vi "Examine clusters.vi"(10 "Cluster centers":string[](array[string]), 11 "Pattern (0) Distance data (1 to X) cluster (X+1) output":string[][](array[string])) -> (1 "position counts":T1[](array[typedef]), 2 "Cluster center graph":cluster{"XY Graph":cluster{dbl[], dbl[]}}[](array[cluster]), 3 "Cluster graph":cluster{"XY Graph":cluster{dbl[], dbl[]}[]}[](array[cluster]))   [LabVIEW 2013]
uses:
  cluster.ctl
panel:
  out "Array 2":dbl[](array[numeric])
  out "Cluster":T2
  out "XY Graph 4":cluster{dbl[], dbl[]}(graph)
  in  "XY Graph 6":cluster{dbl[], dbl[]}(graph)
  out "array 2":dbl[][][](array[numeric])
  in  "XY Graph 3":cluster{dbl[], dbl[]}[](graph)
  out "XY Graph":cluster{"X":dbl[], "Y":dbl[]}(graph)
  out "XY Graph 2":cluster{dbl[], dbl[]}[](graph)
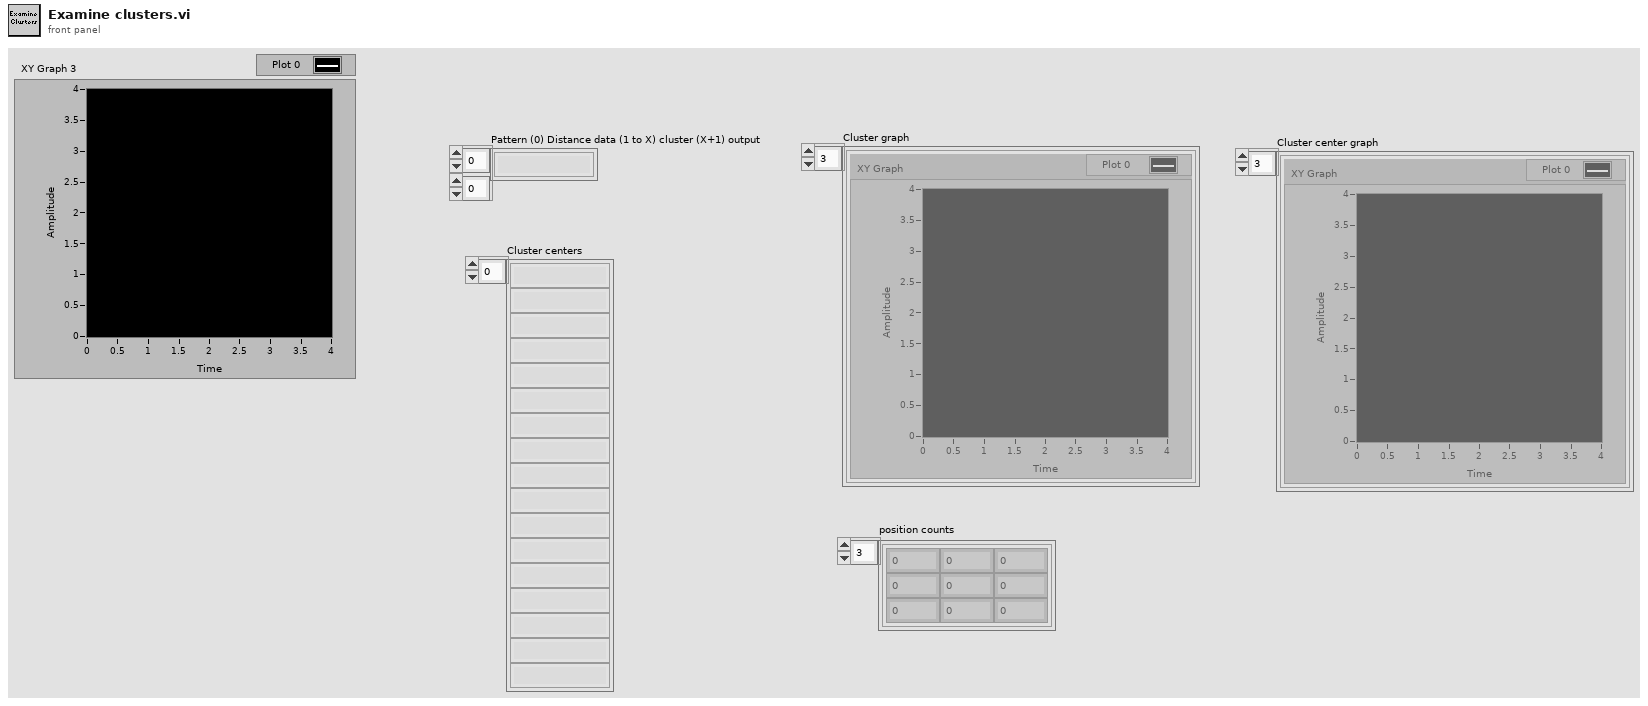
[diagram p1: front panel]
types:
  T1 = typedef "cluster.ctl" = cluster{dbl, dbl, dbl, dbl, dbl, dbl, dbl, dbl, dbl}
  T2 = cluster{dbl, dbl, dbl, dbl, dbl, dbl, dbl, dbl, dbl}
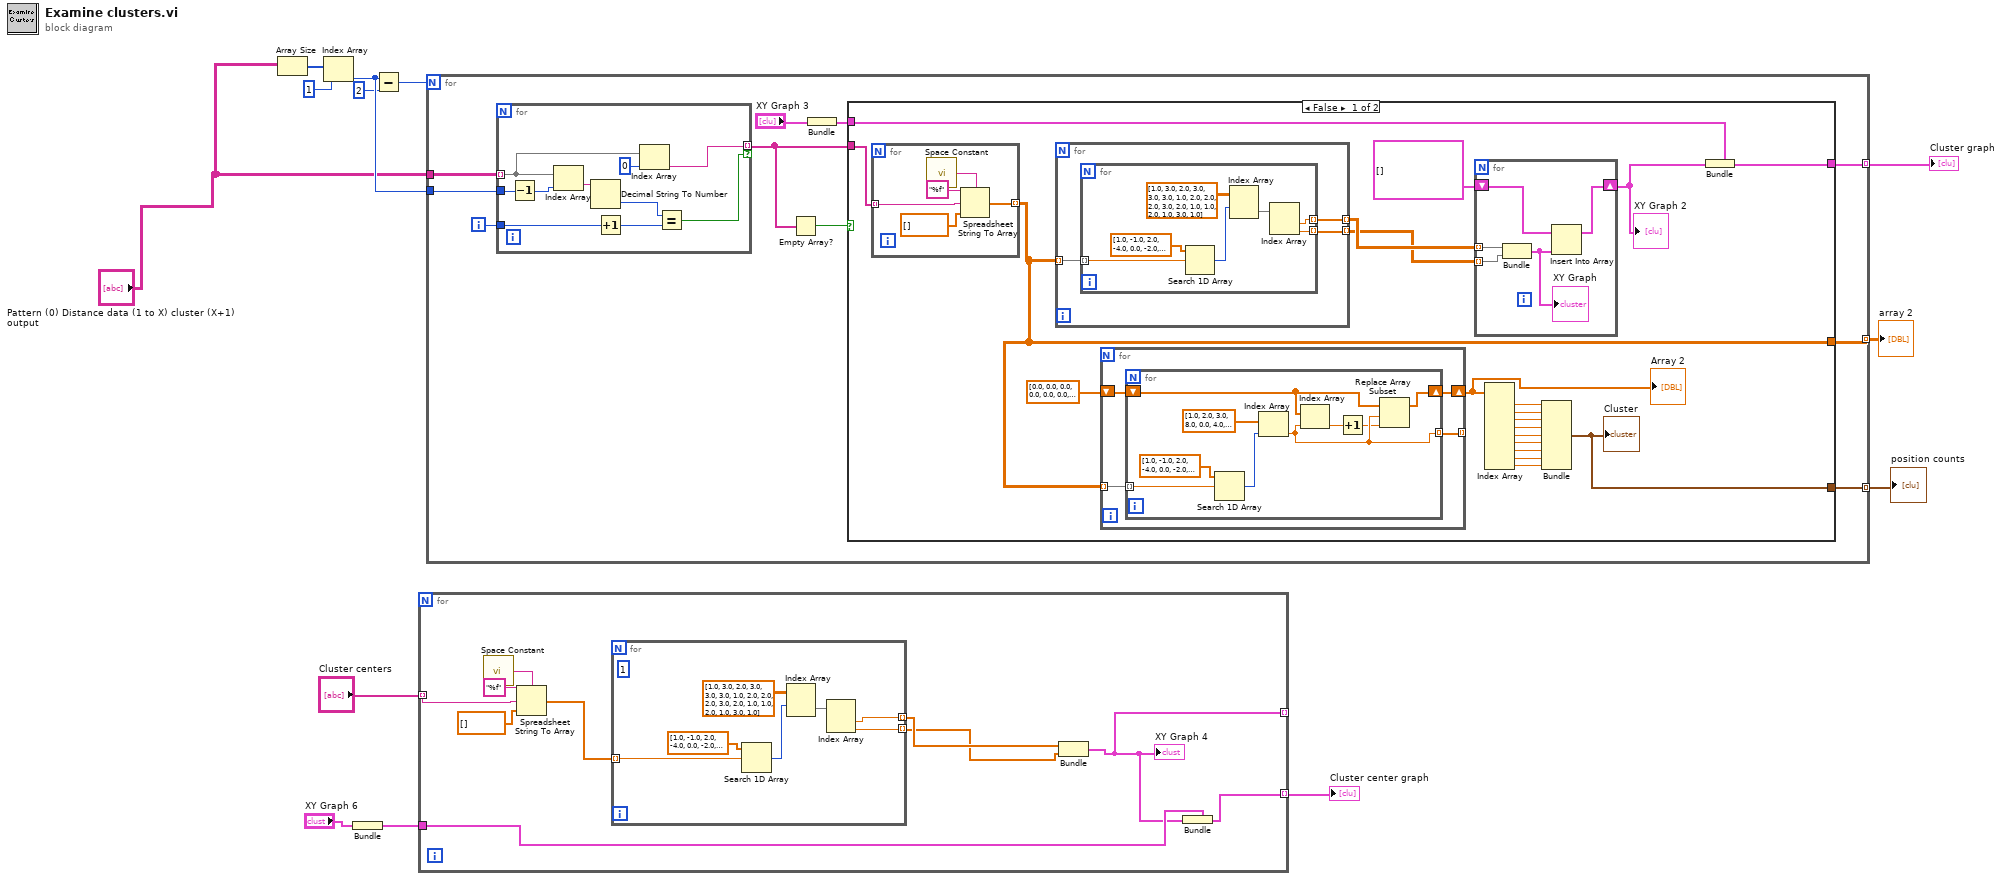
[diagram p0: block diagram]
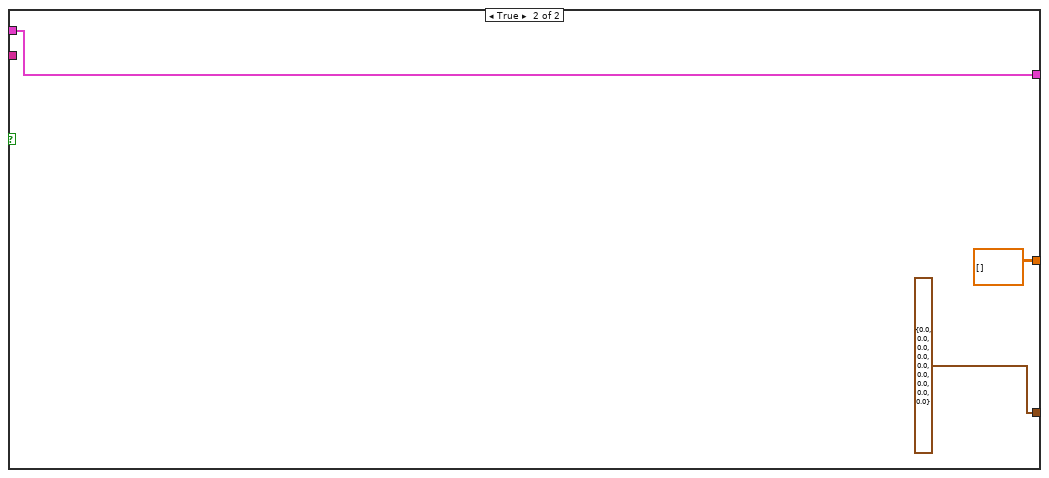
[diagram p2: hidden frame]
diagram:
  n1 = Array Size(array="Pattern (0) Distance data (1 to X) cluster (X+1) output") -> (size(s)=w9:i32[])
  n2 = Index Array(array=w9, index=1) -> (element=w13:i32)
  n3 = Bundle("XY Graph 6"="XY Graph 6") -> (w3:cluster{"XY Graph 6":cluster{dbl[], dbl[]}})  [unwired: 1 in]
  n4 = Subtract(x=w13, y=2) -> (x-y=w12:i32)
  n5 = for {
    tunnel: "Cluster centers" -> [w20] mode=indexing
    tunnel: [w15] -> _ mode=indexing
    tunnel: w3 -> [w16]
    tunnel: [w14] -> w5 mode=indexing
    n6 = call <vilib>:"Space Constant.vi"() -> ("String"=w18:string)
    n7 = Spreadsheet String To Array(delimiter (Tab)=w18, format string="%f", spreadsheet string=w20, array type (2D Dbl)=dbl[] [] ("array 2")) -> (array=w21:dbl[])
    n8 = for {
      tunnel: w21 -> [w30] mode=indexing
      tunnel: [w29] -> w23 mode=indexing
      tunnel: [w28] -> w22 mode=indexing
      (unwired) 1
      n9 = Search 1D Array(1D array=dbl[] [1.0, -1.0, 2.0, -4.0, 0.0, -2.0, 4.0, -3.0, 3.0], element=w30) -> (index of element=w25:i32)  [unwired: 1 in]
      n10 = Index Array(array=dbl[][] [[1.0, 3.0], [2.0, 3.0], [3.0, 3.0], [1.0, 2.0], [2.0, 2.0], [3.0, 2.0], [1.0, 1.0], [2.0, 1.0], [3.0, 1.0]], index (row)=w25) -> (element=w24:dbl[])  [unwired: 1 in]
      n11 = Index Array(array=w24) -> (element #1=w29:dbl, element #2=w28:dbl)  [unwired: 2 in]
    }
    n12 = Bundle(w23, w22) -> (w15:cluster{dbl[], dbl[]})  [unwired: 1 in]
    "XY Graph 4" <- w15
    n13 = Bundle(cluster=w16, "XY Graph 6"=w15) -> (w14:cluster{"XY Graph 6":cluster{dbl[], dbl[]}})
  }
  "Cluster center graph" <- w5
  n14 = for {
    N: w12 -> [_]
    tunnel: "Pattern (0) Distance data (1 to X) cluster (X+1) output" -> [w40]
    tunnel: w13 -> [w39]
    tunnel: [w33] -> w8 mode=indexing
    tunnel: [w32] -> w6 mode=indexing
    tunnel: [w31] -> w1 mode=indexing
    i -> [w38]
    n15 = for {
      tunnel: w40 -> [w103] mode=indexing
      tunnel: w39 -> [w105]
      tunnel: w38 -> [w101]
      tunnel: [w97] -> w37 mode=indexing if=w98
      n16 = Decrement(x=w105) -> (x-1=w106:i32)
      n17 = Index Array(array=w103, index=w106) -> (element=w102:string)
      n18 = Decimal String To Number(string=w102) -> (number=w99:i32)  [unwired: 2 in, 1 out]
      n19 = Increment(x=w101) -> (x+1=w100:i32)
      n20 = Index Array(array=w103, index=0) -> (element=w97:string)
      n21 = Equal?(x=w99, y=w100) -> (x = y?=w98:bool)
    }
    n22 = Empty Array?(array=w37) -> (empty?=w36:bool)
    n23 = Bundle("XY Graph 3"="XY Graph 3") -> (w34:cluster{"XY Graph 3":cluster{dbl[], dbl[]}[]})  [unwired: 1 in]
    n24 = case shown="False" w36 {
      tunnel: w37 -> [w60 _]
      tunnel: w34 -> [w56 w96]
      tunnel: [w55 w96] -> w33
      tunnel: [w41 dbl[][] [] ("array 2")] -> w32
      tunnel: [w42 T2 {0.0, 0.0, 0.0, 0.0, 0.0, 0.0, 0.0, 0.0, 0.0} ("Cluster 2")] -> w31
      frame False {
        n25 = for {
          tunnel: w60 -> [w90] mode=indexing
          tunnel: [w89] -> w41 mode=indexing
          n26 = call <vilib>:"Space Constant.vi"() -> ("String"=w92:string)
          n27 = Spreadsheet String To Array(delimiter (Tab)=w92, format string="%f", spreadsheet string=w90, array type (2D Dbl)=dbl[] [] ("array 2")) -> (array=w89:dbl[])
        }
        n28 = for {
          tunnel: w41 -> [w81] mode=indexing
          tunnel: [w80] -> w58 mode=indexing
          tunnel: [w79] -> w57 mode=indexing
          n29 = for {
            tunnel: w81 -> [w87] mode=indexing
            tunnel: [w84] -> w80 mode=indexing
            tunnel: [w83] -> w79 mode=indexing
            n30 = Search 1D Array(1D array=dbl[] [1.0, -1.0, 2.0, -4.0, 0.0, -2.0, 4.0, -3.0, 3.0], element=w87) -> (index of element=w85:i32)  [unwired: 1 in]
            n31 = Index Array(array=dbl[][] [[1.0, 3.0], [2.0, 3.0], [3.0, 3.0], [1.0, 2.0], [2.0, 2.0], [3.0, 2.0], [1.0, 1.0], [2.0, 1.0], [3.0, 1.0]], index (row)=w85) -> (element=w82:dbl[])  [unwired: 1 in]
            n32 = Index Array(array=w82) -> (element #1=w84:dbl, element #2=w83:dbl)  [unwired: 2 in]
          }
        }
        n33 = for {
          tunnel: w41 -> [w64] mode=indexing
          tunnel: [w63] -> _ mode=indexing
          shift-right: [w61] -> w43
          shift-left: dbl[] [0.0, 0.0, 0.0, 0.0, 0.0, 0.0, 0.0, 0.0, 0.0] -> [w62]
          n34 = for {
            tunnel: w64 -> [w73] mode=indexing
            tunnel: [w67] -> w63 mode=indexing
            shift-right: [w65] -> w61
            shift-left: w62 -> [w68]
            n35 = Search 1D Array(1D array=dbl[] [1.0, -1.0, 2.0, -4.0, 0.0, -2.0, 4.0, -3.0, 3.0], element=w73) -> (index of element=w72:i32)  [unwired: 1 in]
            n36 = Index Array(array=dbl[] [1.0, 2.0, 3.0, 8.0, 0.0, 4.0, 7.0, 6.0, 5.0], index=w72) -> (element=w67:dbl)
            n37 = Index Array(array=w68, index=w67) -> (element=w69:dbl)
            n38 = Increment(x=w69) -> (x+1=w66:dbl)
            n39 = Replace Array Subset(array=w68, new element=w66, index=w67) -> (w65:dbl[])
          }
        }
        "Array 2" <- w43
        n40 = for {
          tunnel: w58 -> [w78] mode=indexing
          tunnel: w57 -> [w77] mode=indexing
          shift-right: [w75] -> w54
          shift-left: cluster{dbl[], dbl[]}[] [] -> [w76]
          n41 = Bundle(w78, w77) -> (w74:cluster{dbl[], dbl[]})  [unwired: 1 in]
          "XY Graph" <- w74
          n42 = Insert Into Array(array=w76, new element=w74) -> (w75:cluster{dbl[], dbl[]}[])  [unwired: 1 in]
        }
        "XY Graph 2" <- w54
        n43 = Index Array(array=w43) -> (element #1=w44:dbl, element #2=w45:dbl, element #3=w46:dbl, element #4=w47:dbl, element #5=w48:dbl, element #6=w49:dbl, element #7=w50:dbl, element #8=w51:dbl, element #9=w52:dbl)  [unwired: 9 in]
        n44 = Bundle(w44, w45, w46, w47, w48, w49, w50, w51, w52) -> (w42:T2)  [unwired: 1 in]
        "Cluster" <- w42
        n45 = Bundle(cluster=w56, "XY Graph 3"=w54) -> (w55:cluster{"XY Graph 3":cluster{dbl[], dbl[]}[]})
      }
      frame True {
      }
    }
  }
  "Cluster graph" <- w8
  "array 2" <- w6
  "position counts" <- w1
